vi "solar_excel Worksheet Create.vi"(8 "error in (no error)":errorcluster, 10 "New Worksheet Name":string, 11 "Excel Workbook":T1) -> (0 "error out":errorcluster, 3 "Excel Worksheet":T2)   [LabVIEW 2018]
doc: "This creates a new Worksheet in the Workbook and returns the Worksheet reference."
uses:
  solar_excel_ctl Worksheet.ctl
  solar_excel_ctl TSV.ctl
  solar_excel_ctl Workbook.ctl
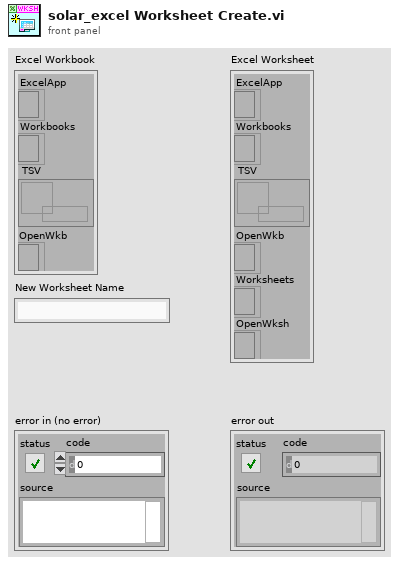
[diagram p1: front panel]
types:
  T1 = typedef "solar_excel_ctl Workbook.ctl" = cluster{"ExcelApp":refnum<k7>, "Workbooks":refnum<k7>, "TSV":refnum<queue>, "OpenWkb":refnum<k7>}
  T2 = typedef "solar_excel_ctl Worksheet.ctl" = cluster{"ExcelApp":refnum<k7>, "Workbooks":refnum<k7>, "TSV":refnum<queue>, "OpenWkb":refnum<k7>, "Worksheets":refnum<k7>, "OpenWksh":refnum<k7>}
  T3 = typedef "solar_excel_ctl TSV.ctl" = cluster{"Path":path, "Dirty":bool, "ActiveSheet":u8, "Worksheets":string[], "Worksheet Cells":cluster{"Cells":string[][]}[]}
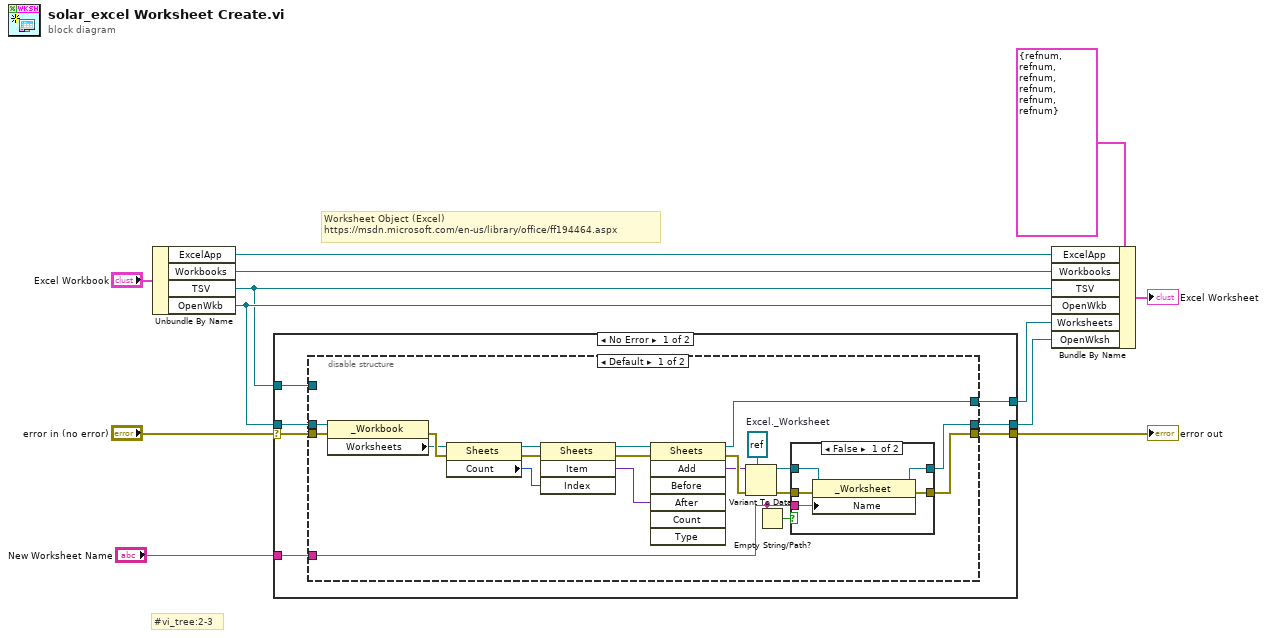
[diagram p0: block diagram]
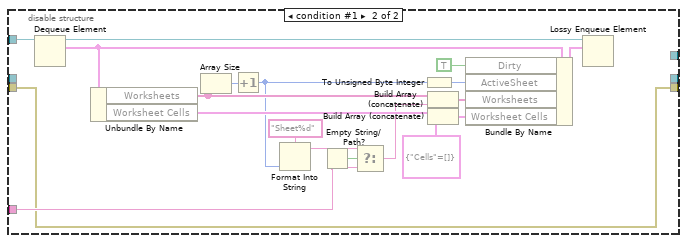
[diagram p3: hidden frame]
diagram:
  # "#vi_tree:2-3"
  # "Worksheet Object (Excel)\nhttps://msdn.microsoft.com/en-us/library/office/ff194464.aspx"
  n1 = Unbundle By Name("Excel Workbook") -> ("ExcelApp"=w8:refnum<k7>, "Workbooks"=w7:refnum<k7>, "TSV"=w1:refnum<queue>, "OpenWkb"=w6:refnum<k7>)
  n2 = case shown="No Error" "error in (no error)" {
    selector: "error in (no error)" -> [w19 w66]
    tunnel: [w17 w66] -> w12
    tunnel: w6 -> [w18 _]
    tunnel: [w14 _] -> w4
    tunnel: [w16 _] -> w3
    tunnel: "New Worksheet Name" -> [w15 _]
    tunnel: w1 -> [w13 _]
    frame No Error {
      n3 = disable-structure shown="Default" {
        disable-tunnel: w19 -> [w39 w54]
        disable-tunnel: w18 -> [w37 _]
        disable-tunnel: [w34 w54] -> w17
        disable-tunnel: [w32 _] -> w16
        disable-tunnel: w15 -> [w22 w57]
        disable-tunnel: [w20 _] -> w14
        disable-tunnel: w13 -> [_ w65]
        frame condition #0 (active) {
          w35 = refnum<k7> refnum  # Excel._Worksheet
          n4 = property class="_Workbook"(reference=w37, error in=w39) -> (error out=w38:errorcluster, "Worksheets"=w30:refnum<k7>)  [unwired: 1 out]
          n5 = property class="Sheets"(reference=w30, error in=w38) -> (reference out=w29:refnum<k7>, error out=w31:errorcluster, "Count"=w28:i32)
          n6 = invoke class="Sheets" method="Item"(reference=w29, error in=w31, "Index"=w28) -> (reference out=w26:refnum<k7>, error out=w27:errorcluster, "Item"=w25:variant)  [unwired: 1 in, 1 out]
          n7 = invoke class="Sheets" method="Add"(reference=w26, error in=w27, "After"=w25) -> (reference out=w20:refnum<k7>, error out=w24:errorcluster, "Add"=w23:variant)  [unwired: 4 in, 4 out]
          n8 = Variant To Data(error in=w24, type=w35, Variant=w23) -> (data=w33:refnum<k7>, error out=w36:errorcluster)
          n9 = Empty String/Path?(string/path=w22) -> (empty?=w21:bool)
          n10 = case shown="False" w21 {
            tunnel: w36 -> [w44 w46]
            tunnel: [w43 w46] -> w34
            tunnel: w33 -> [w42 w45]
            tunnel: [w41 w45] -> w32
            tunnel: w22 -> [w40 _]
            frame False {
              n11 = property class="_Worksheet"(reference=w42, error in=w44, "Name"=w40) -> (reference out=w41:refnum<k7>, error out=w43:errorcluster)
            }
            frame True {
            }
          }
        }
        frame condition #1 {
          n12 = Dequeue Element(queue=w65) -> (queue out=w64:refnum<queue>, element=w63:T3)  [unwired: 2 in, 2 out]
          n13 = Unbundle By Name(w63) -> ("Worksheets"=w52:string[], "Worksheet Cells"=w61:cluster{"Cells":string[][]}[])
          n14 = Array Size(array=w52) -> (size(s)=w51:i32)
          n15 = Increment(x=w51) -> (x+1=w50:i32)
          n16 = Format Into String(format string="Sheet%d", w50) -> (resulting string=w47:string)  [unwired: 2 in, 1 out]
          n17 = Empty String/Path?(string/path=w57) -> (empty?=w58:bool)
          n18 = Select(t=w47, s=w58, f=w57) -> (s? t:f=w55:string)
          n19 = To Unsigned Byte Integer(number=w50) -> (unsigned 8bit integer=w49:u8)
          n20 = Build Array (concatenate)(w52, w55) -> (w59:string[])
          n21 = Build Array (concatenate)(w61, cluster{"Cells":string[][]} {"Cells"=[]} ("element")) -> (w60:cluster{"Cells":string[][]}[])
          n22 = Bundle By Name(cluster=w63, "Dirty"=TRUE, "ActiveSheet"=w49, "Worksheets"=w59, "Worksheet Cells"=w60) -> (w62:T3)
          n23 = Lossy Enqueue Element(queue=w64, element=w62) -> ()  [unwired: 1 in, 4 out]
        }
      }
    }
    frame Error {
    }
  }
  "error out" <- w12
  n24 = Bundle By Name(cluster=T2 {"ExcelApp"=refnum, "Workbooks"=refnum, "TSV"=refnum, "OpenWkb"=refnum, "Worksheets"=refnum, "OpenWksh"=refnum} ("Excel Worksheet 2"), "ExcelApp"=w8, "Workbooks"=w7, "TSV"=w1, "OpenWkb"=w6, "Worksheets"=w4, "OpenWksh"=w3) -> (→"Excel Worksheet":T2)
